vi "Camera Control.vi"(5 "Error":string, 6 "Height":i32, 7 "Width":i32, 8 "Image Pointer":i32, 9 "Operation":i8) -> (0 "Height":i32, 1 "Width":i32, 2 "Image Pointer":i32, 3 "Operation":i8, 4 "Error":string)   [LabVIEW 2011, in "labvvis.lvlib"]
doc: "Copies a single frame from the first available sequence grabber to the image specified."
uses:
  <userlib>/labvvis/labvvis.lvlib
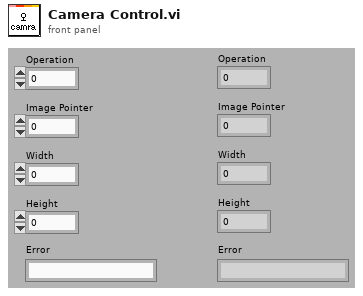
[diagram p1: front panel]
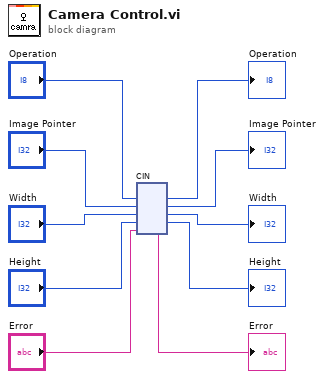
[diagram p0: block diagram]
diagram:
  n1 = cin("Operation", "Image Pointer", "Width", "Height", "Error") -> (→"Operation":i8, →"Image Pointer":i32, →"Width":i32, →"Height":i32, →"Error":string)
